vi "Write To Csv Test.vi"() -> ()   [LabVIEW 2021, in "Test Files.lvlib"]
uses:
  Test Files.lvlib
  <vilib>/addons/_JKI Toolkits/Caraya/classes/Test/Test.lvclass
  <vilib>/addons/_JKI Toolkits/Caraya/classes/Assert/Assert.lvclass
  CustomSortPath.lvlib
  <vilib>/addons/_JKI Toolkits/Caraya/classes/Assert/Assert Equal Value_Variant.vi
panel:
  out "error out":errorcluster
  in  "error in (no error)":errorcluster
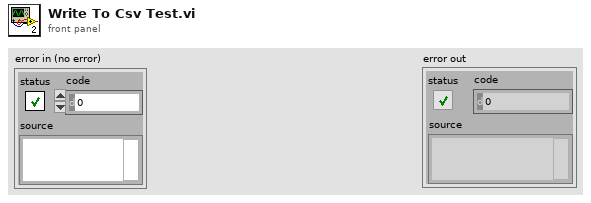
[diagram p1: front panel]
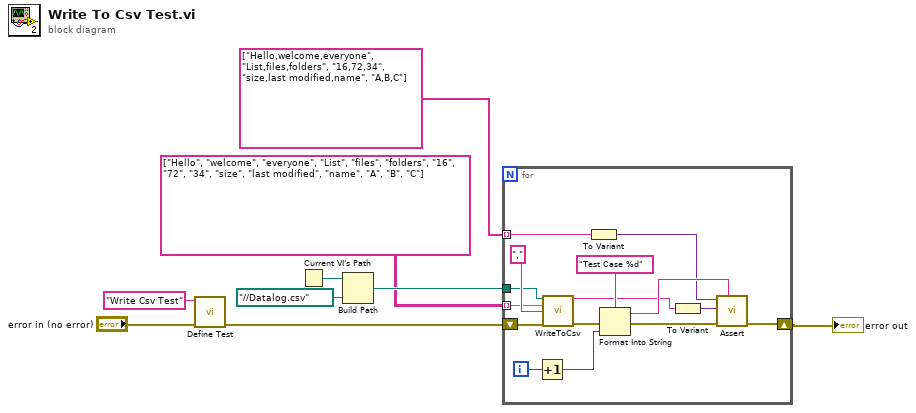
[diagram p0: block diagram]
diagram:
  n1 = call <vilib>:"Define Test.vi"("error in (no error)"="error in (no error)", "Label (VI Title)"="Write Csv Test") -> ("error out"=w7:errorcluster)  [unwired: 8 in, 1 out]
  n2 = Current VI's Path() -> (path=w6:path)
  n3 = Build Path(base path=w6, name or relative path=path "../../Datalog.csv") -> (appended path=w4:path)
  n4 = for {
    tunnel: w4 -> [w22]
    tunnel: string[][] [["Hello", "welcome", "everyone"], ["List", "files", "folders"], ["16", "72", "34"], ["size", "last modified", "name"], ["A", "B", "C"]] ("appended array") -> [w21] mode=indexing
    tunnel: string[] ["Hello,welcome,everyone", "List,files,folders", "16,72,34", "size,last modified,name", "A,B,C"] -> [w19] mode=indexing
    shift-right: [w11] -> w1
    shift-left: w7 -> [w23]
    i -> [w16]
    n5 = Increment(x=w16) -> (x+1=w15:i32)
    n6 = call "WriteToCsv.vi"("File Path"=w22, "StringArray"=w21, "delimiter (Tab)"=",", "error in (no error)"=w23) -> ("String Out"=w10:string, "error out"=w20:errorcluster)  [unwired: 10 in]
    n7 = To Variant(anything=w19) -> (Variant=w13:variant)
    n8 = Format Into String(format string="Test Case %d", error in=w20, w15) -> (resulting string=w14:string, error out=w18:errorcluster)  [unwired: 1 in]
    n9 = To Variant(anything=w10) -> (Variant=w12:variant)
    n10 = call-poly <vilib>:"Assert.vi"("Label"=w14, "error in (no error)"=w18, "Y"=w12, "X"=w13) -> ("error out"=w11:errorcluster)  [unwired: 6 in, 1 out]
  }
  "error out" <- w1
